vi "Actor.vi"(11 "Class":refnum<class "DAQmx - Analog Output Single Sample.lvclass">) -> ()   [LabVIEW 2021, in "DAQmx - Analog Output Single Sample.lvclass"]
uses:
  DAQmx - Analog Output Single Sample.lvclass
  C:/TSA/DAQmx-Bus/Source/DAQmx-Bus.lvclass
  DAQmx-Bus.lvclass/DAQmx-Bus.ctl
  DAQmx - Analog Output Single Sample.lvclass/DAQmx - Analog Output Single Sample.ctl
  Properties/Read DAQmx Task.vi
  Properties/Read timeout.vi
  Properties/Read Values DVR.vi
  Properties/Read Stop.vi
  Properties/Read Sync.vi
  <vilib>/DAQmx/miscellaneous.llb/DAQmx Fill In Error Info.vi
  <vilib>/DAQmx/write.llb/DAQmx Write (Analog 1D DBL NChan 1Samp).vi
  <vilib>/platform/TimedLoop/XDataNode/XDataNode.xnode
  <vilib>/Platform/TimedLoop/XDataNode/nitl_modes.ctl
  <vilib>/Platform/TimedLoop/XDataNode/XDNodeRunTimeDep.lvlib
  <vilib>/Platform/TimedLoop/XDataNode/wakeup.ctl
  <vilib>/Platform/TimedLoop/XDataNode/timing_clust.ctl
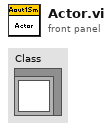
[diagram p1: front panel]
types:
  T1 = typedef "XDNodeRunTimeDep.lvlib/timing_clust.ctl" = cluster{"Expected End [f-1]":u64, "Actual End [f-1]":u64, "Finished Late? [f-1]":bool, "Expected End [i-1]":u64, "Actual End [i-1]":u64, "Finished Late? [i-1]":bool, "Expected Start [i]":u64, "Actual Start [i]":u64, "Expected Start [f]":u64, "Actual Start [f]":u64, "Source Name":string, "Structure Name":string, "Period":i64, "Deadline":i64, "Offset":i64, "Start":i64, "Priority":i32, "Timeout":i32, "Mode":T2, "Wakeup Reason":T3, "Error":errorcluster, "Source Type":string, "Secondary Source Type":string, "Global End Time":u64, "Global Start Time":u64, "Frame Duration":u64, "Iteration Duration":u64, "Assigned CPU":i32, "I/O Scan Engine Mode":u32}
  T2 = typedef "XDNodeRunTimeDep.lvlib/nitl_modes.ctl" = enum32{"No Change", "Process missed periods, maintain original phase", "Discard missed periods, maintain original phase", "Process missed periods, ignore original phase", "Discard missed periods, ignore original phase"}
  T3 = typedef "XDNodeRunTimeDep.lvlib/wakeup.ctl" = enum32{"Normal", "Aborted", "Asynchronous wakeup", "Timing source error", "Timed loop error", "Timeout"}
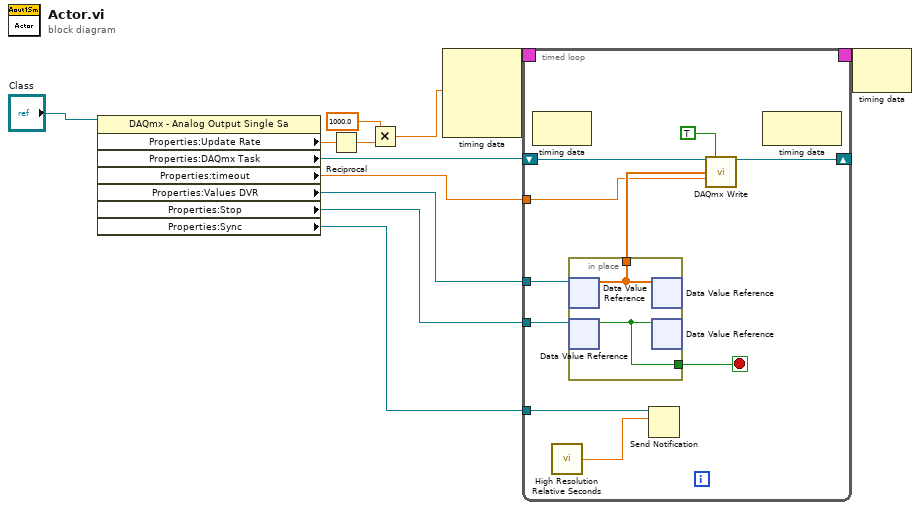
[diagram p0: block diagram]
diagram:
  n1 = property class="DAQmx - Analog Output Single Sa"(reference="Class") -> ("Properties:Update Rate"=w4:dbl, "Properties:DAQmx Task"=w7:refnum<k21>, "Properties:timeout"=w11:dbl, "Properties:Values DVR"=w10:refnum<data-value>, "Properties:Stop"=w12:refnum<data-value>, "Properties:Sync"=w8:refnum<notifier>)  [unwired: 1 in, 2 out]
  n2 = Reciprocal(x=w4) -> (1/x=w3:dbl)
  n3 = Multiply(x=1000.0, y=w3) -> (x*y=w1:dbl)
  n4 = node-c288(w1) -> (w6:T1)  [unwired: 3 in]
  n5 = timed-loop {
    shift-right: [w16] -> _
    shift-left: w7 -> [w17]
    tunnel: w12 -> [w22]
    tunnel: w11 -> [w14]
    tunnel: w10 -> [w20]
    tunnel: w8 -> [w18]
    timing: w6 -> [_]
    timing-out: [_] -> w5
    stop <- w21 stop-if-true
    n6 = node-c288() -> ()  [unwired: 1 in, 1 out]
    n7 = call <vilib>:"High Resolution Relative Seconds.vi"() -> ("relative seconds"=w19:dbl)
    n8 = in-place {
      in-place-border: [w26] -> w21
      in-place-border: [w25] -> w15
      n9 = in-place-dvr #1(w20) -> (w25:dbl[])  [unwired: 1 out]
      n10 = in-place-dvr #2(w22) -> (w26:bool)  [unwired: 1 out]
      n11 = in-place-dvr #1(w25) -> ()  [unwired: 2 out]
      n12 = in-place-dvr #2(w26) -> ()  [unwired: 2 out]
    }
    n13 = Send Notification(notification=w19, notifier=w18) -> ()  [unwired: 1 in, 2 out]
    n14 = call-poly <vilib>:"DAQmx Write.vi"("task/channels in"=w17, "auto start"=TRUE, "data"=w15, "timeout"=w14) -> ("task out"=w16:refnum<k21>)  [unwired: 9 in, 2 out]
    n15 = node-c288() -> ()  [unwired: 1 in, 1 out]
  }
  n16 = node-c288(w5) -> ()  [unwired: 1 out]
